vi "Open_Config.vi"   [LabVIEW 2019]
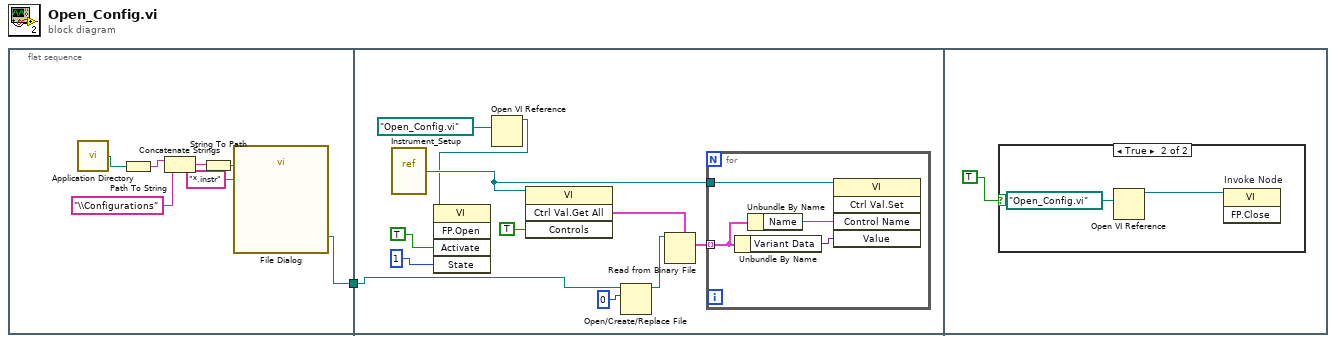
[diagram p0: block diagram]
diagram:
  n1 = flat-sequence {
    tunnel: [w2] -> w1
    tunnel: w1 -> [w14]
    frame #0 {
      n2 = call <vilib>:"Application Directory.vi"() -> ("Application Directory"=w8:path)
      n3 = Path To String(path=w8) -> (string=w7:string)
      n4 = Concatenate Strings(w7, "\\Configurations") -> (w5:string)
      n5 = String To Path(string=w5) -> (path=w4:path)
      n6 = call "File Dialog"("start path"=w4, "pattern (all files)"="*.instr") -> ("selected path"=w2:path)  [unwired: 10 in, 3 out]
    }
    frame #1 {
      n7 = vi-ref "Instrument_Setup.vi"() -> (w11:refnum<vi>)
      n8 = Open VI Reference(vi path=path "Open_Config.vi") -> (vi reference=w9:refnum<vi>)  [unwired: 5 in, 1 out]
      n9 = invoke class="VI" method="FP.Open"(reference=w9, "Activate"=TRUE, "State"=1) -> ()  [unwired: 2 in, 5 out]
      n10 = invoke class="VI" method="Ctrl Val.Get All"(reference=w11, "Controls"=TRUE) -> ("Get All Control Values Variant"=w15:cluster{"Name":string, "Variant Data":variant}[])  [unwired: 2 in, 3 out]
      n11 = Open/Create/Replace File(file path (use dialog)=w14, operation (0:open)=0) -> (refnum out=w17:refnum<file>)  [unwired: 4 in, 2 out]
      n12 = Read from Binary File(5:w15, 11:w17) -> (2:w16:cluster{"Name":string, "Variant Data":variant}[])  [unwired: 4 in, 3 out]
      n13 = for {
        tunnel: w11 -> [w23]
        tunnel: w16 -> [w20] mode=indexing
        n14 = Unbundle By Name(w20) -> ("Variant Data"=w21:variant)
        n15 = Unbundle By Name(w20) -> ("Name"=w22:string)
        n16 = invoke class="VI" method="Ctrl Val.Set"(reference=w23, "Control Name"=w22, "Value"=w21) -> ()  [unwired: 2 in, 5 out]
      }
    }
    frame #2 {
      n17 = case shown="True" TRUE {
        frame False {
        }
        frame True {
          n18 = Open VI Reference(vi path=path "Open_Config.vi") -> (vi reference=w25:refnum<vi>)  [unwired: 5 in, 1 out]
          n19 = invoke on="Invoke Node" class="VI" method="FP.Close"(reference=w25) -> ()  [unwired: 2 in, 3 out]
        }
      }
    }
  }
